vi "Find Pockels calibration for wavelength.vi"(8 "error in (no error)":errorcluster, 11 "Wav":dbl) -> (0 "error out":errorcluster, 3 "Ok ?":bool)   [LabVIEW 2020]
uses:
  Globals/gl_Calibration globals.vi
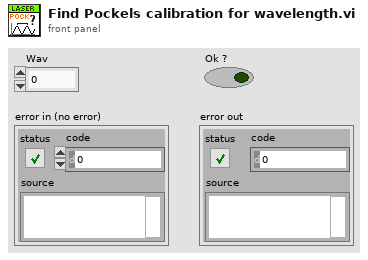
[diagram p1: front panel]
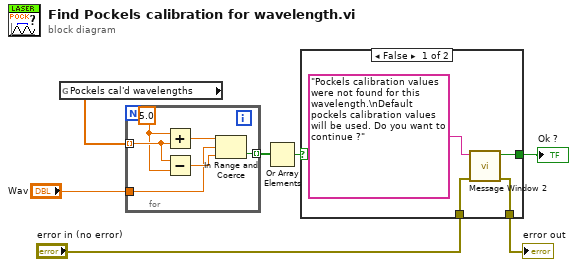
[diagram p0: block diagram]
diagram:
  n1 = global read "gl_Calibration globals.vi" "Pockels cal'd wavelengths"() -> (w1:dbl[])
  n2 = for {
    tunnel: w1 -> [w9] mode=indexing
    tunnel: "Wav" -> [w11]
    tunnel: [w10] -> w2 mode=indexing
    w8 = 5.0 ("x")
    n3 = Add(x=w8, y=w9) -> (x+y=w13:dbl)
    n4 = Subtract(x=w9, y=w8) -> (x-y=w12:dbl)
    n5 = In Range and Coerce(upper limit=w13, x=w11, lower limit=w12) -> (In Range?=w10:bool)  [unwired: 1 out]
  }
  n6 = Or Array Elements(Boolean array=w2) -> (logical OR=w3:bool)
  n7 = case shown="False" w3 {
    selector: w3 -> [_ w19]
    tunnel: [w16 w19] -> w4
    tunnel: "error in (no error)" -> [w15 w18]
    tunnel: [w14 w18] -> w6
    frame False {
      n8 = call "Message Window 2.vi"("error in (no error)"=w15, "Message string"="Pockels calibration values were not found for this wavelength.\nDefault pockels calibration values will be used. Do you want to continue ?") -> ("error out (no error)"=w14:errorcluster, "Ok ?"=w16:bool)  [unwired: 8 in]
    }
    frame True {
    }
  }
  "error out" <- w6
  "Ok ?" <- w4
